vi "Copy .LLB to NI VeriStand dir.vi"(5 "Files Generated by Build":path[](array[path]), 6 "Top Level/Always Included VIs":path[](array[path]), 7 "Destination Path":path, 8 "error in (no error)":errorcluster, 9 "Target Name":string, 10 "Build Specification Name":string, 11 "Project Path":path) -> (0 "error out":errorcluster)   [LabVIEW 2024]
doc: "This VI is called after each run of a build specification. The VI will copy the generated LLB (Engine or System Explorer) into the VeriStand Custom Device folder (...\\Documents\\National Instruments\\NI VeriStand 2013...)."
uses:
  NationalInstruments.VeriStand
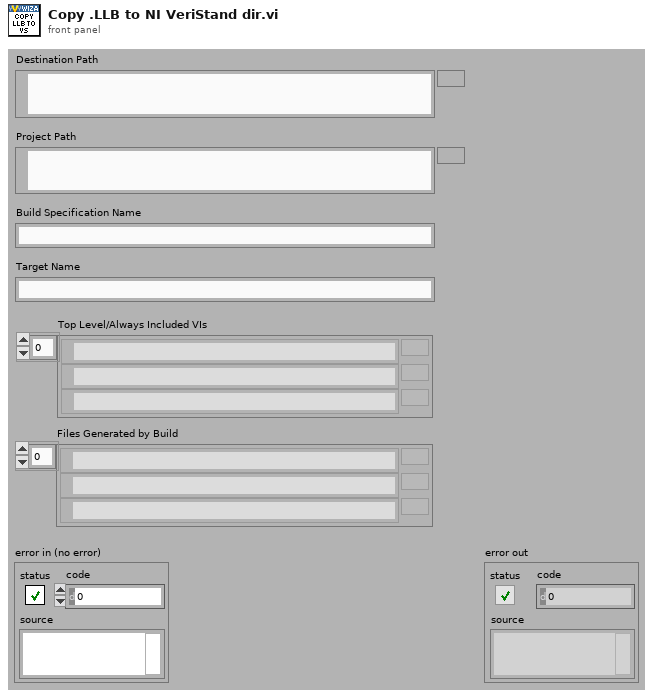
[diagram p1: front panel]
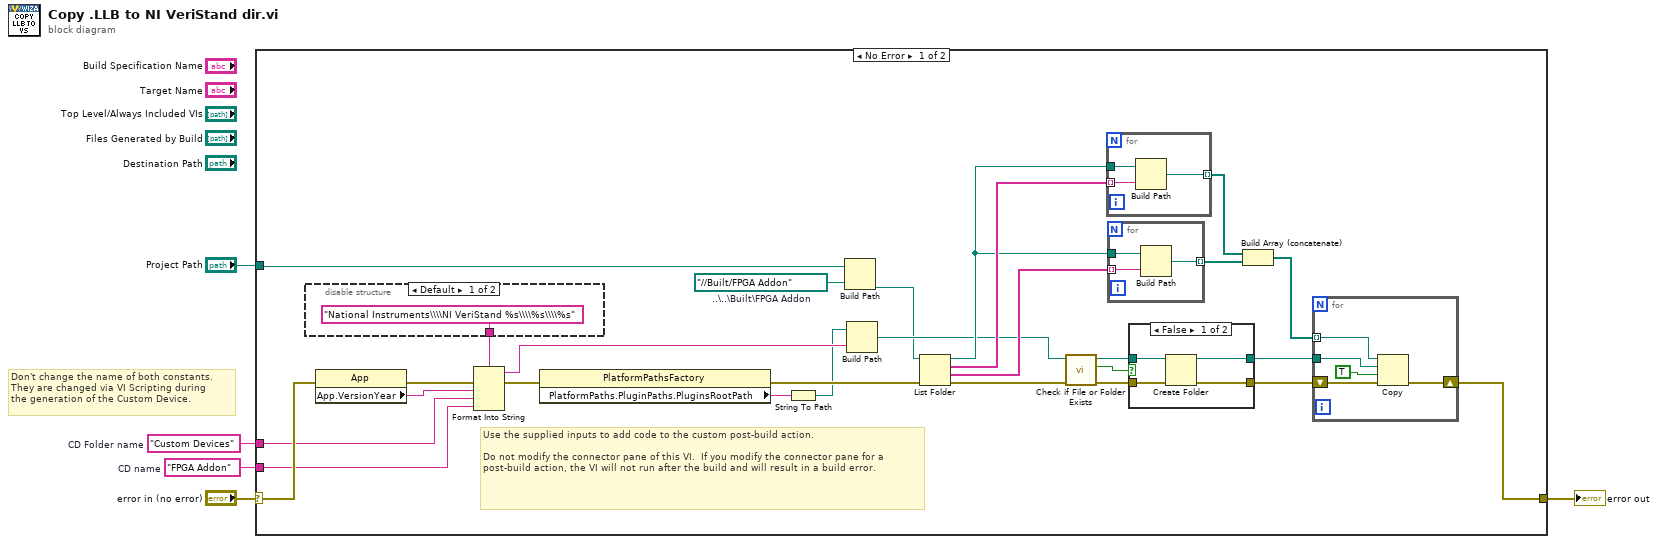
[diagram p0: block diagram]
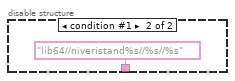
[diagram p2: hidden frame]
diagram:
  w1 = "FPGA Addon"  # CD name
  w2 = "Custom Devices"  # CD Folder name
  # "Don't change the name of both constants.\nThey are changed via VI Scripting during\nthe generation of the Custom Device."
  n1 = case shown="No Error" "error in (no error)" {
    selector: "error in (no error)" -> [w18 w53]
    tunnel: [w20 w53] -> w3
    tunnel: "Project Path" -> [w17 _]
    tunnel: w2 -> [w13 _]
    tunnel: w1 -> [w11 _]
    frame No Error {
      w10 = path "../../Built/FPGA Addon"  # ..\..\Built\FPGA Addon
      # "Use the supplied inputs to add code to the custom post-build action.\n\nDo not modify the connector pane of this VI.  If you modify the connector pane for a post-build action, the VI will not run after the build and will result in a build error."
      n2 = disable-structure shown="Default" {
        disable-tunnel: ["National Instruments\\\\NI VeriStand %s\\\\%s\\\\%s" ("name or relative path") "lib64//niveristand%s//%s//%s" ("name or relative path")] -> w12
        frame condition #0 (active) {
        }
        frame condition #1 {
        }
      }
      n3 = property class="App"(error in=w18) -> (error out=w22:errorcluster, "App.VersionYear"=w21:string)  [unwired: 1 in, 1 out]
      n4 = Format Into String(format string=w12, error in=w22, w21, w13, w11) -> (resulting string=w23:string, error out=w8:errorcluster)  [unwired: 1 in]
      n5 = property class="PlatformPathsFactory"(error in=w8) -> (error out=w9:errorcluster, "PlatformPaths.PluginPaths.PluginsRootPath"=w7:string)  [unwired: 1 in, 1 out]
      n6 = String To Path(string=w7) -> (path=w6:path)
      n7 = Build Path(base path=w17, name or relative path=w10) -> (appended path=w14:path)
      n8 = Build Path(base path=w6, name or relative path=w23) -> (appended path=w19:path)
      n9 = List Folder(path=w14, error in=w9) -> (path out=w26:path, filenames=w33:string[], folder names=w27:string[], error out=w24:errorcluster)  [unwired: 2 in]
      n10 = call <vilib>:"Check if File or Folder Exists.vi"("error in (no error)"=w24, "path"=w19) -> ("error out"=w28:errorcluster, "file or folder exists?"=w30:bool, "dup path"=w29:path)  [unwired: 7 in]
      n11 = for {
        tunnel: w33 -> [w51] mode=indexing
        tunnel: w26 -> [w52]
        tunnel: [w50] -> w32 mode=indexing
        n12 = Build Path(base path=w52, name or relative path=w51) -> (appended path=w50:path)
      }
      n13 = for {
        tunnel: w27 -> [w48] mode=indexing
        tunnel: w26 -> [w49]
        tunnel: [w47] -> w25 mode=indexing
        n14 = Build Path(base path=w49, name or relative path=w48) -> (appended path=w47:path)
      }
      n15 = case shown="False" w30 {
        tunnel: w29 -> [w39 w41]
        tunnel: w28 -> [w38 w40]
        tunnel: [w37 w41] -> w16
        tunnel: [w36 w40] -> w15
        frame False {
          n16 = Create Folder(path (use dialog)=w39, error in=w38) -> (created path=w37:path, error out=w36:errorcluster)  [unwired: 1 in, 1 out]
        }
        frame True {
        }
      }
      n17 = Build Array (concatenate)(w32, w25) -> (w31:path[])
      n18 = for {
        tunnel: w31 -> [w43] mode=indexing
        shift-right: [w44] -> w20
        shift-left: w15 -> [w45]
        tunnel: w16 -> [w42]
        n19 = Copy(8:w45, 9:TRUE ("overwrite (F)"), 10:w42, 11:w43) -> (0:w44:errorcluster)  [unwired: 1 in, 2 out]
      }
    }
    frame Error {
    }
  }
  "error out" <- w3
